vi "app1.vi"() -> ()   [LabVIEW 2013]
uses:
  <vilib>/Utility/miscctls.llb/LVPointTypeDef.ctl
panel:
  in  "Listbox":i32(listbox)
  in  "Slide":dbl(slide)=2.3024830699774266 scale=0.0..10.0
  out "XY Graph":cluster{"X":dbl, "Y":dbl}[](graph)
  in  "Knob 5":dbl(knob) scale=0.0..10.0
  in  "Knob 4":dbl(knob) scale=0.0..10.0
  in  "Knob 3":dbl(knob) scale=0.0..10.0
  in  "Knob 2":dbl(knob) scale=0.0..10.0
  in  "Knob":dbl(knob) scale=0.0..10.0
  in  "stop":bool
  # "App Foo Bar"
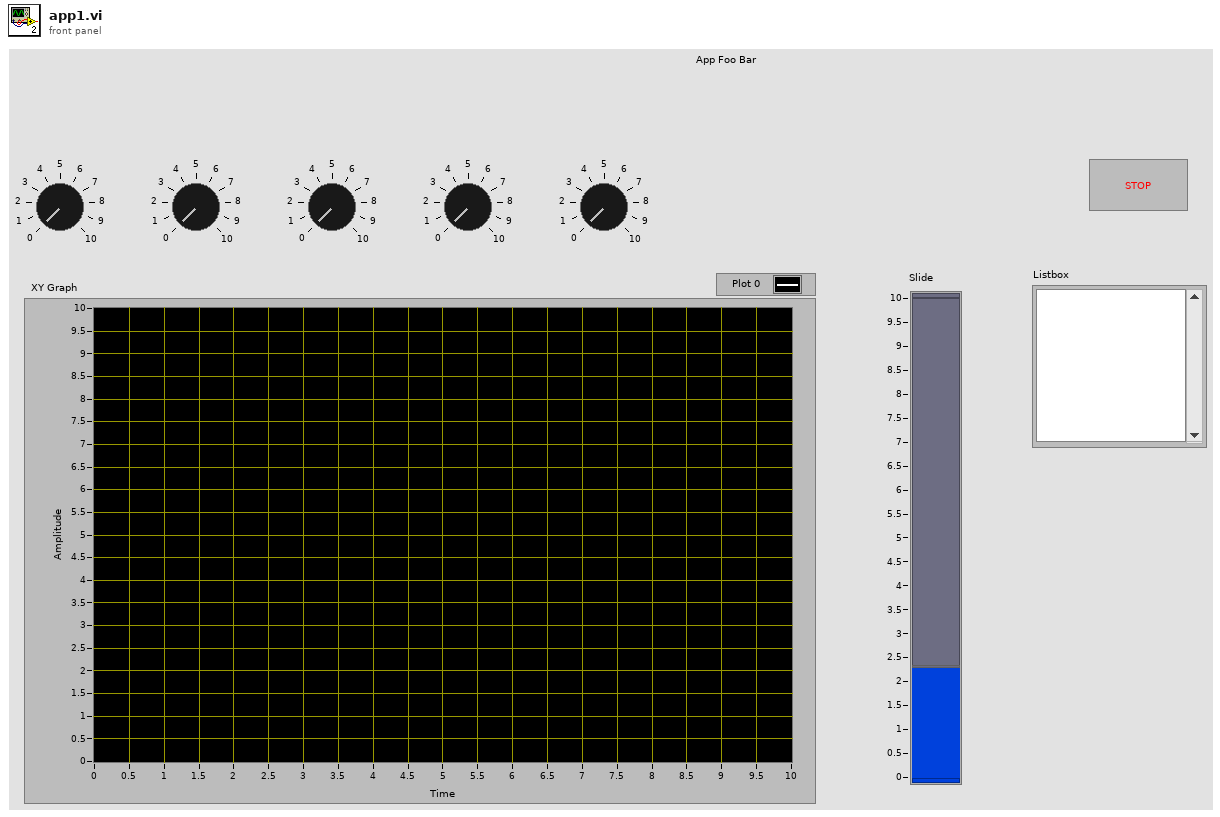
[diagram p1: front panel]
types:
  T1 = typedef "LVPointTypeDef.ctl" = cluster{"Horizontal":i16, "Vertical":i16}
  T2 = typedef "LVAllMonitorsDisplayTypeDef.ctl" = cluster{"Bounds":cluster{"Left":i16, "Top":i16, "Right":i16, "Bottom":i16}, "Depth":i16}[]
  T3 = typedef "LVRectTypeDef.ctl" = cluster{"Left":i16, "Top":i16, "Right":i16, "Bottom":i16}
  T4 = cluster{"Bounds":cluster{"Left":i16, "Top":i16, "Right":i16, "Bottom":i16}, "Depth":i16}
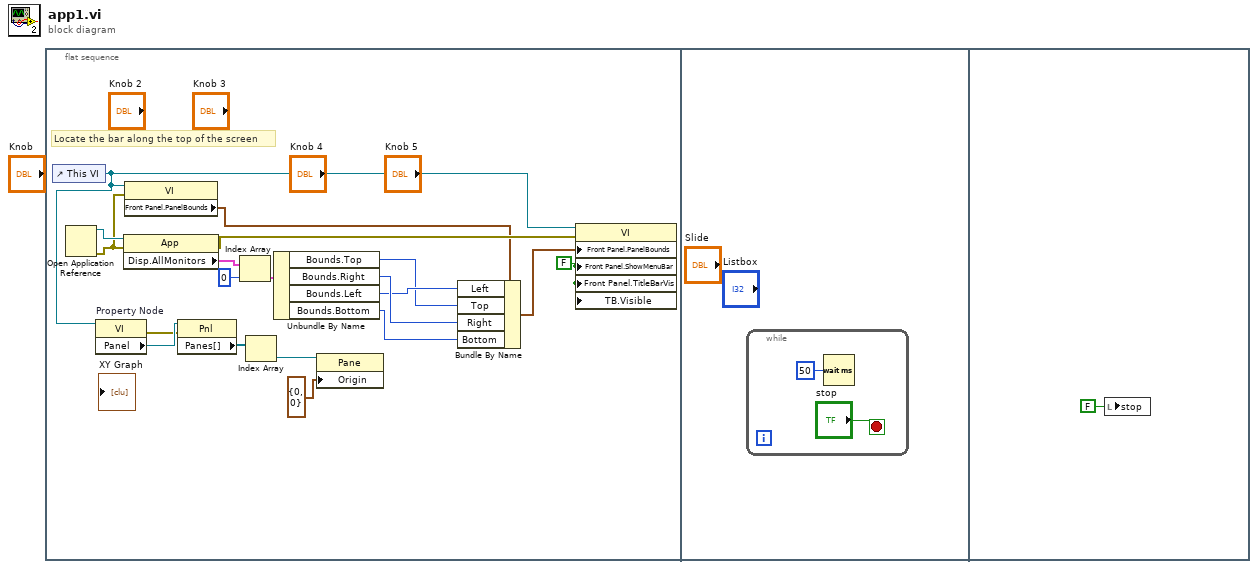
[diagram p0: block diagram]
diagram:
  n1 = flat-sequence {
    frame #0 {
      w3 = FALSE ("Front Panel Window:Show Menu Bar")
      # "Locate the bar along the top of the screen"
      n2 = control-ref of="This VI"() -> (w4:refnum<vi>)
      n3 = Open Application Reference() -> (0:w11:errorcluster, 3:w12:refnum<vi>)  [unwired: 4 in]
      n4 = property on="Property Node" class="VI"(reference=w4) -> (error out=w8:errorcluster, "Panel"=w9:refnum<vi>)  [unwired: 1 in, 1 out]
      n5 = property class="App"(reference=w12, error in=w11) -> (error out=w16:errorcluster, "Disp.AllMonitors"=w18:T2)  [unwired: 1 out]
      n6 = property class="VI"(reference=w4, error in=w11) -> ("Front Panel.PanelBounds"=w10:T3)  [unwired: 2 out]
      n7 = property class="Pnl"(reference=w9, error in=w8) -> ("Panes[]"=w7:refnum<vi>[])  [unwired: 2 out]
      n8 = Index Array(array=w18, index=0) -> (element=w19:T4)
      n9 = Index Array "Index Array"(array=w7) -> (element=w6:refnum<vi>)  [unwired: 1 in]
      n10 = Unbundle By Name(w19) -> ("Bounds.Top"=w2:i16, "Bounds.Right"=w14:i16, "Bounds.Left"=w13:i16, "Bounds.Bottom"=w1:i16)
      n11 = property class="Pane"(reference=w6, "Origin"=T1 {"Horizontal"=0, "Vertical"=0}) -> ()  [unwired: 1 in, 2 out]
      n12 = Bundle By Name(cluster=w10, "Left"=w13, "Top"=w2, "Right"=w14, "Bottom"=w1) -> (w15:T3)
      n13 = property on="Property Node" class="VI"(reference=w4, error in=w16, "Front Panel.PanelBounds"=w15, "Front Panel.ShowMenuBar"=w3, "Front Panel.TitleBarVis"=w3, "TB.Visible"=w3) -> ()  [unwired: 2 out]
    }
    frame #1 {
      n14 = while {
        stop <- "stop" stop-if-true
        n15 = Wait (ms)(milliseconds to wait=u32 50) -> ()  [unwired: 1 out]
      }
    }
    frame #2 {
      n16 = local write "stop"(FALSE ("stop")) -> ()
    }
  }
